vi "Create CircularBuffer ByVar.vi"(5 "Buffer Name":string, 7 "CircularBuffer in":refnum<class "CircularBuffer.lvclass">, 8 "error in (no error)":errorcluster, 9 "Type":variant, 11 "BufferSize":u32=1) -> (0 "error out":errorcluster, 2 "Buffer name created":string, 3 "CircularBuffer out":refnum<class "CircularBuffer.lvclass">)   [LabVIEW 2016, in "CircularBuffer.lvclass"]
uses:
  CircularBuffer.lvclass
  types/type/type.lvclass
  types/type.U8/type.U8.lvclass
  Typedefs/BufferSize.ctl
  types/type.DBL/type.DBL.lvclass
  <vilib>/Utility/VariantDataType/VariantType.lvlib
  I:/levy_SVN/lockin/branches/jlevy/HAL-Webinar-master/Subsystems/CircularBuffer/types/type/type.lvclass
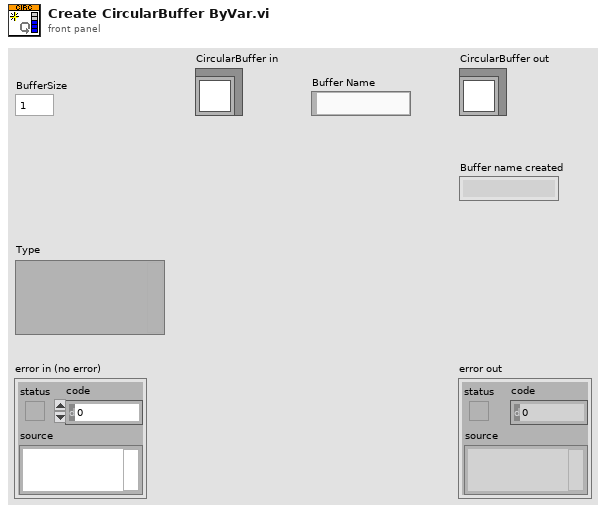
[diagram p1: front panel]
types:
  T1 = typedef "CircularBuffer.lvclass/BufferSize.ctl" = u32
  T2 = typedef "VariantType.lvlib/Type.ctl" = enum8{"Invalid Type", "Void", "I8", "I16", "I32", "I64", "U8", "U16", "U32", "U64", "Single Float", "Double Float", "Extended Float", "Single Complex", "Double Complex", "Extended Complex", "Enum U8", "Enum U16", "Enum U32", "Enum U64", "Single Float With Unit", "Double Float With Unit", "Extended Float With Unit", "Single Complex with Unit", "Double Complex with Unit", "Extended Complex with Unit", "Boolean", "String", "Path", "Picture", "Tag", "Array", "Cluster", "Variant", "LV Variant", "Waveform", "Timestamp", "Digital Waveform", "Digital Data", "ExpressData", "Refnum", "External Data", "VI", "Poly VI", "LabVIEW Class Instance", "Fixed Point"}
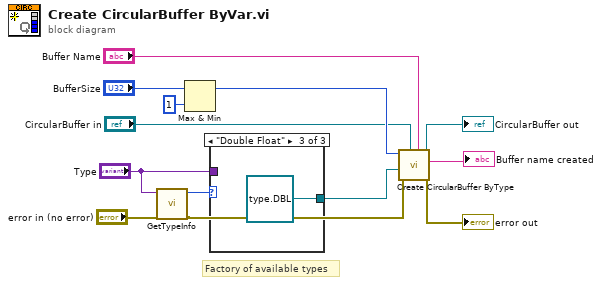
[diagram p0: block diagram]
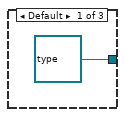
[diagram p2: hidden frame]
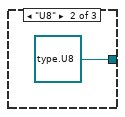
[diagram p3: hidden frame]
diagram:
  # "Factory of available types"
  n1 = call <vilib>:"GetTypeInfo.vi"("error in (no error)"="error in (no error)", "Variant"="Type") -> ("error out"=w2:errorcluster, "Type Enum"=w1:T2)  [unwired: 5 in, 3 out]
  n2 = Max & Min(x="BufferSize", y=T1 1) -> (max(x,y)=w11:T1)  [unwired: 1 out]
  n3 = case shown="\"Double Float\"" w1 {
    tunnel: "Type" -> [_ _ _]
    tunnel: [refnum<class "type.lvclass"> refnum ("type.lvclass") refnum<class "type.U8.lvclass"> refnum ("type.U8.lvclass") refnum<class "type.DBL.lvclass"> refnum ("type.DBL.lvclass")] -> w5
    frame Default {
    }
    frame "U8" {
    }
    frame "Double Float" {
    }
  }
  n4 = call "Create CircularBuffer ByType.vi"("Buffer Name"="Buffer Name", "CircularBuffer in"="CircularBuffer in", "error in (no error)"=w2, "type"=w5, "BufferSize"=w11) -> ("error out"=→"error out":errorcluster, "Buffer name created"=→"Buffer name created":string, "CircularBuffer out"=→"CircularBuffer out":refnum<class "CircularBuffer.lvclass">)  [unwired: 4 in]
